vi "(SubVI) Delete Force offset of xDNA and Force.vi"(0 "Force":dbl[](array[numeric]), 1 "Upper Force (pN)":dbl, 2 "xDNA":dbl[](array[numeric]), 3 "force constant":dbl, 4 "Lower Force (pN)":dbl, 5 "Set lower foce offset?":bool) -> (6 "cut-full Force":dbl[](array[numeric]), 8 "cut-full xDNA":dbl[](array[numeric]))   [LabVIEW 2014]
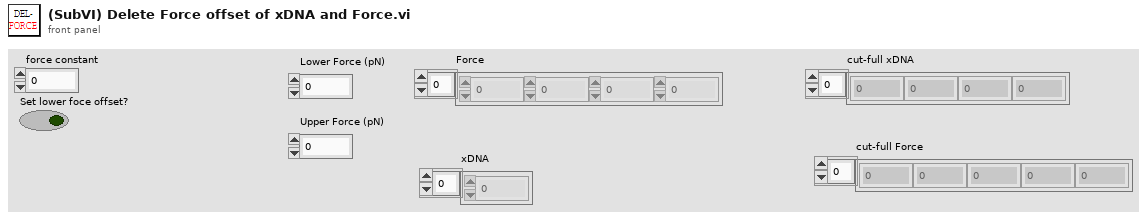
[diagram p1: front panel]
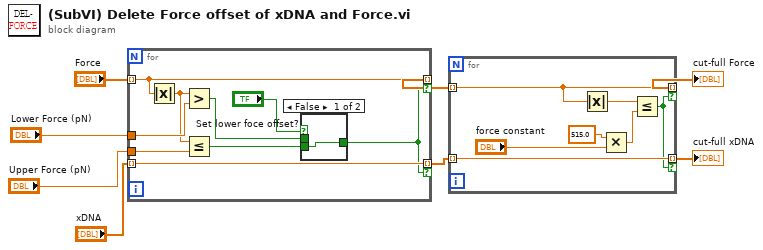
[diagram p0: block diagram]
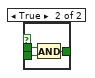
[diagram p2: hidden frame]
diagram:
  n1 = for {
    tunnel: "Force" -> [w16] mode=indexing
    tunnel: [w16] -> w5 mode=indexing if=w10
    tunnel: "Lower Force (pN)" -> [w13]
    tunnel: "xDNA" -> [w17] mode=indexing
    tunnel: [w17] -> w4 mode=indexing if=w10
    tunnel: "Upper Force (pN)" -> [w11]
    n2 = Absolute Value(x=w16) -> (abs(x)=w12:dbl)
    n3 = Greater?(x=w12, y=w13) -> (0:w14:bool)
    n4 = Less Or Equal?(x=w12, y=w11) -> (x <= y?=w15:bool)
    n5 = case shown="False" "Set lower foce offset?" {
      tunnel: w15 -> [w18 w21]
      tunnel: w14 -> [_ w20]
      tunnel: [w18 w19] -> w10
      frame False {
      }
      frame True {
        n6 = And(x=w20, y=w21) -> (x .and. y?=w19:bool)
      }
    }
  }
  n7 = for {
    tunnel: w5 -> [w23] mode=indexing
    tunnel: [w23] -> w3 mode=indexing if=w24
    tunnel: [w28] -> w2 mode=indexing if=w24
    tunnel: w4 -> [w28] mode=indexing
    n8 = Absolute Value(x=w23) -> (abs(x)=w22:dbl)
    n9 = Multiply(x=515.0, y="force constant") -> (x*y=w25:dbl)
    n10 = Less Or Equal?(x=w22, y=w25) -> (x <= y?=w24:bool)
  }
  "cut-full Force" <- w3
  "cut-full xDNA" <- w2
